vi "common_generate_app_message.vi"(8 "error in (no error)":errorcluster, 11 "event data":T1) -> (0 "error out":errorcluster)   [LabVIEW 2019]
doc: "Generates an app-wide event to <b>event data</b> to another module. \n\nIf the framework hasn't been initialized, then Error 1 thrown when trying to generate the event. This error is caught and cleared in this VI. Use common_global_app_event_fgv.vi with action \"init\" to initialize framework."
uses:
  common data types/common_event_data.ctl
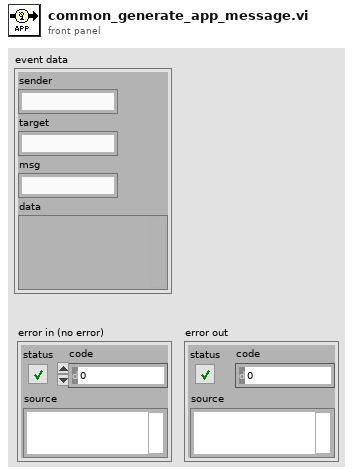
[diagram p1: front panel]
types:
  T1 = typedef "common_event_data.ctl" = cluster{"sender":string, "target":string, "msg":string, "data":variant}
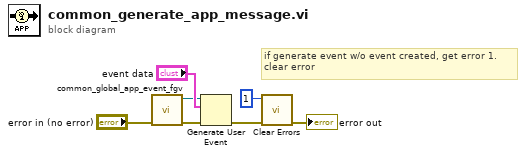
[diagram p0: block diagram]
diagram:
  # "if generate event w/o event created, get error 1. \nclear error"
  n1 = call "common_global_app_event_fgv.vi"("error in (no error)"="error in (no error)") -> ("error out"=w7:errorcluster, "app event"=w4:refnum<user-event>)  [unwired: 9 in]
  n2 = Generate User Event(user event=w4, event data cluster="event data", error in=w7) -> (error out=w2:errorcluster)  [unwired: 1 in, 1 out]
  n3 = call <vilib>:"Clear Errors.vi"("error in (no error)"=w2, "specific error code to clear (0: all)"=1) -> ("error out"=→"error out":errorcluster)  [unwired: 4 in, 1 out]
